vi "FABR-Process Frame.vi"(0 "Runtime in":T2, 7 "SCL in":cluster{T1[]}[](array[cluster]), 9 "AI Waveforms":dbl[](array[numeric]), 11 "error in (no error)":errorcluster, 12 "Reject":dbl, 13 "override":bool) -> (2 "reject fraction":dbl, 3 "Raw":dbl[](array[numeric]), 4 "Runtime out":T2, 8 "SCL out":cluster{T1[]}[](array[cluster]), 10 "update":T1[](array[typedef]), 15 "error out":errorcluster)   [LabVIEW 2020]
uses:
  Typedefs/FABR-Runtime Data.ctl
  Typedefs/FABR-Stimulus Ticket.ctl
  Typedefs/FABR-Stimulus Condition.ctl
  <vilib>/Analysis/baseanly.llb/Mean.vi
  <vilib>/Analysis/baseanly.llb/Mean (DBL).vi
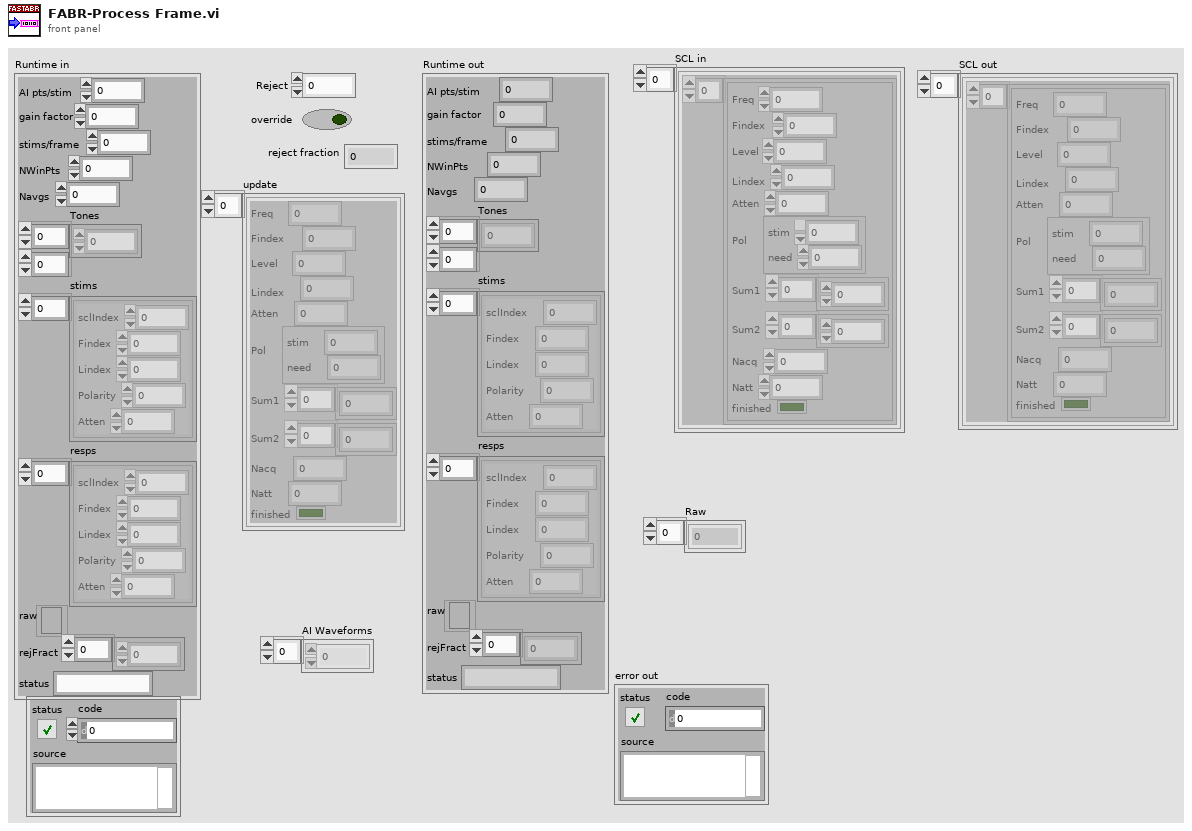
[diagram p1: front panel]
types:
  T1 = typedef "FABR-Stimulus Condition.ctl" = cluster{"Freq":dbl, "Findex":i32, "Level":dbl, "Lindex":i32, "Atten":dbl, "Pol":cluster{"stim":i32, "need":i32}, "Sum1":dbl[], "Sum2":dbl[], "Nacq":i32, "Natt":i32, "finished":bool}
  T2 = typedef "FABR-Runtime Data.ctl" = cluster{"AI pts/stim":i32, "gain factor":dbl, "stims/frame":i32, "NWinPts":i32, "Navgs":i32, "Tones":dbl[][], "stims":T3[], "resps":T3[], "raw":refnum<file>, "rejFract":dbl[], "status":string}
  T3 = typedef "FABR-Stimulus Ticket.ctl" = cluster{"sclIndex":i32, "Findex":i32, "Lindex":i32, "Polarity":i32, "Atten":dbl}
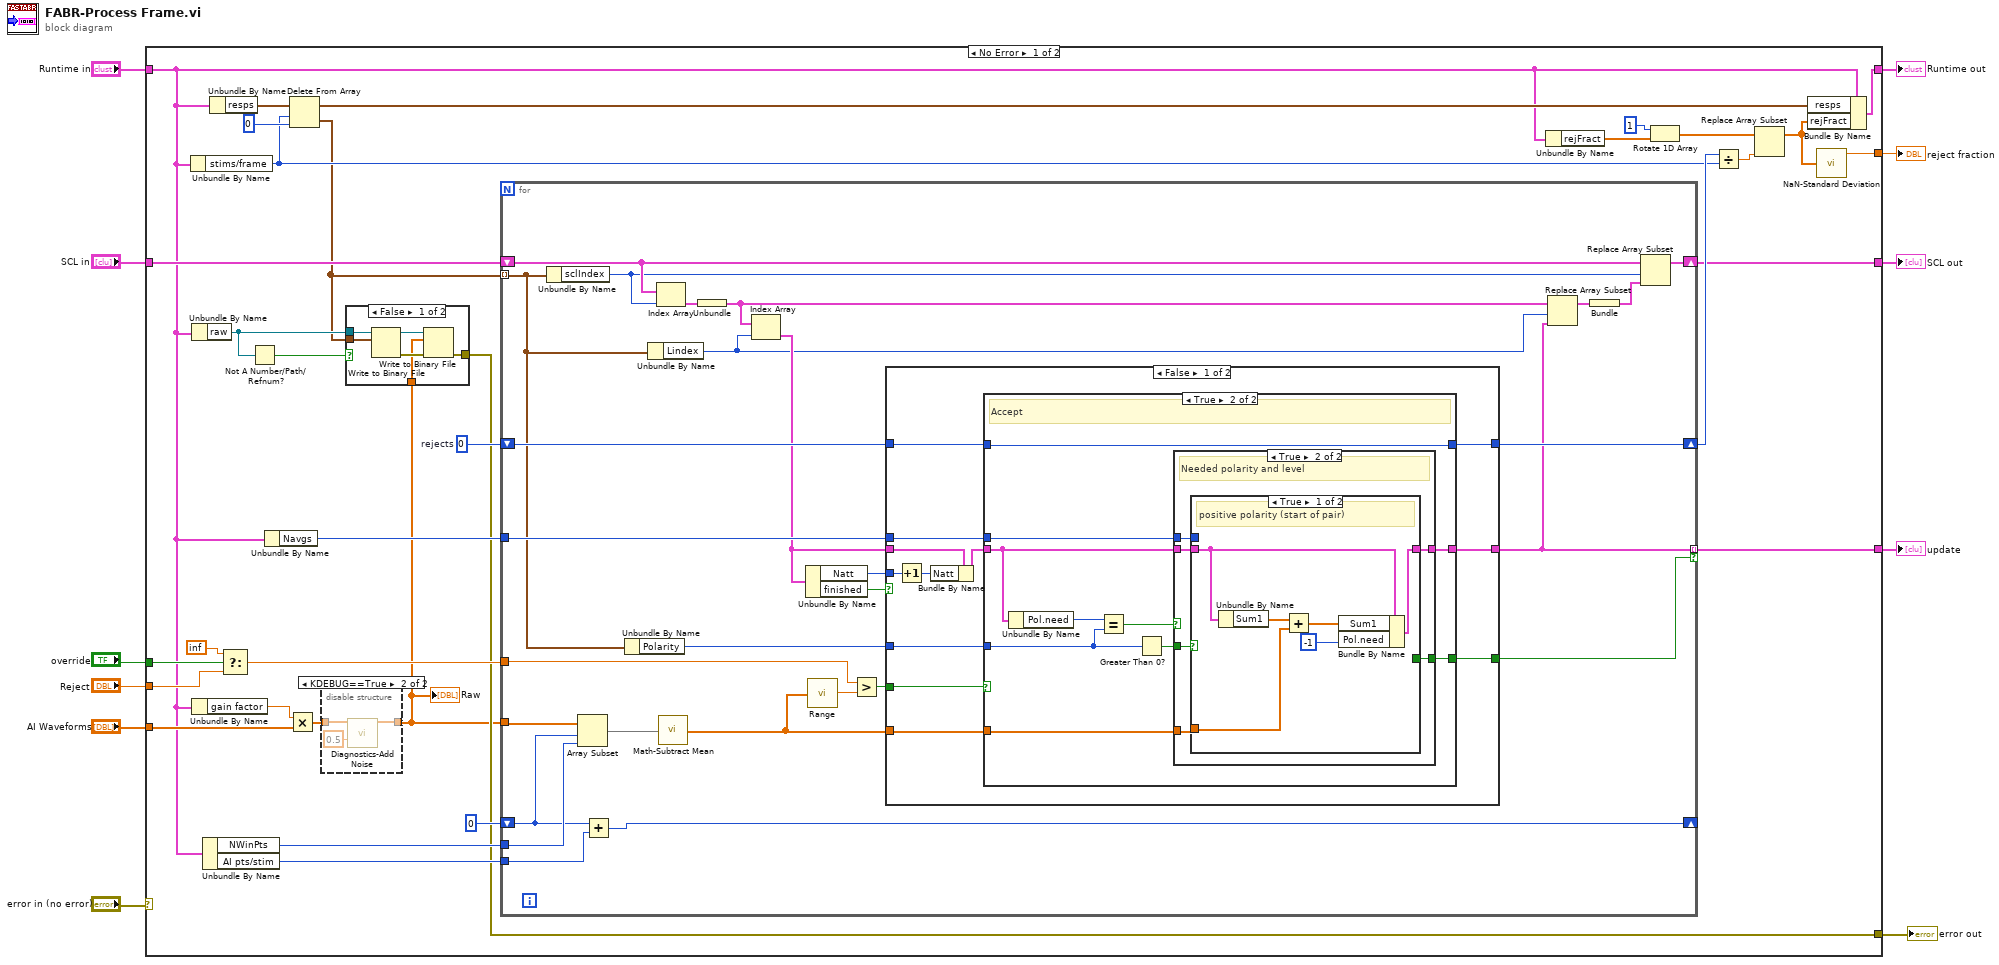
[diagram p0: block diagram]
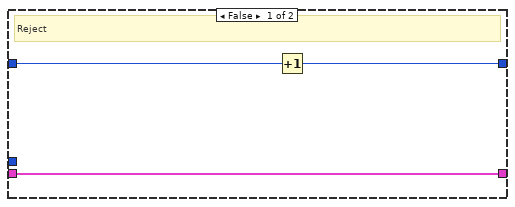
[diagram p4: hidden frame]
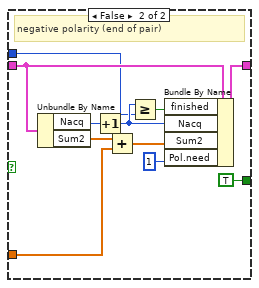
[diagram p6: hidden frame]
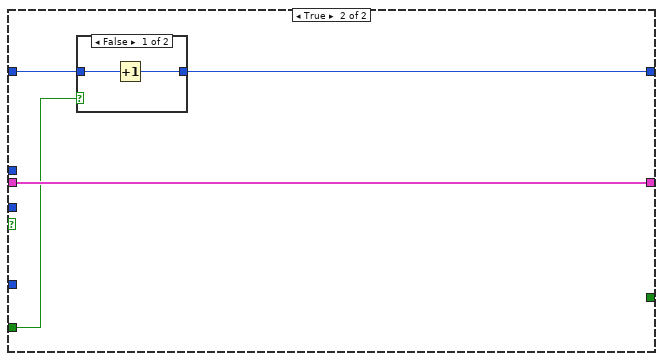
[diagram p7: hidden frame]
diagram:
  n1 = case shown="No Error" "error in (no error)" {
    selector: "error in (no error)" -> [_ w140]
    tunnel: "Runtime in" -> [w20 w139]
    tunnel: "AI Waveforms" -> [w44 _]
    tunnel: "override" -> [w39 _]
    tunnel: "Reject" -> [w38 _]
    tunnel: "SCL in" -> [w31 _]
    tunnel: [w33 _] -> w7
    tunnel: [w32 _] -> w3
    tunnel: [w21 w140] -> w6
    tunnel: [w29 w139] -> w2
    tunnel: [w12 _] -> w1
    frame No Error {
      w35 = 0  # rejects
      n2 = Unbundle By Name(w20) -> ("stims/frame"=w26:i32)
      n3 = Unbundle By Name(w20) -> ("raw"=w23:refnum<file>)
      n4 = Unbundle By Name(w20) -> ("gain factor"=w43:dbl)
      n5 = Unbundle By Name(w20) -> ("NWinPts"=w41:i32, "AI pts/stim"=w40:i32)
      n6 = Unbundle By Name(w20) -> ("resps"=w28:T3[])
      n7 = Select(t=inf, s=w39, f=w38) -> (s? t:f=w36:dbl)
      n8 = Not A Number/Path/Refnum?(number/path/refnum=w23) -> (NaN/Path/Refnum?=w24:bool)
      n9 = Unbundle By Name(w20) -> ("Navgs"=w30:i32)
      n10 = Multiply(x=w43, y=w44) -> (x*y=w17:dbl[])
      n11 = Delete From Array(array=w28, length=w26, index=0) -> (deleted portion=w22:T3[], array with subset deleted=w25:T3[])
      n12 = disable-structure shown="KDEBUG==True" {
        disable-tunnel: w17 -> [w45 w48]
        disable-tunnel: [w45 w47] -> w16
        frame condition #0 (active) {
        }
        frame condition #1 {
          n13 = call "Diagnostics-Add Noise.vi"("Signal"=w48, "Noise RMS"=0.5) -> ("Signal + Noise"=w47:dbl[])  [unwired: 13 in]
        }
      }
      "Raw" <- w16
      n14 = case shown="False" w24 {
        tunnel: w23 -> [w54 _]
        tunnel: w22 -> [w53 _]
        tunnel: w16 -> [w50 _]
        tunnel: [w49 _] -> w21
        frame False {
          n15 = Write to Binary File(file (use dialog)=w54, data=w53) -> (refnum out=w52:refnum<file>, error out=w51:errorcluster)  [unwired: 4 in, 1 out]
          n16 = Write to Binary File(file (use dialog)=w52, data=w50, error in=w51) -> (error out=w49:errorcluster)  [unwired: 3 in, 2 out]
        }
        frame True {
        }
      }
      n17 = for {
        tunnel: w16 -> [w82]
        shift-right: [w78] -> _
        shift-left: 0 -> [w80]
        tunnel: w41 -> [w81]
        tunnel: w40 -> [w79]
        tunnel: w36 -> [w75]
        shift-right: [w72] -> w34
        shift-left: w35 -> [w71]
        shift-right: [w68] -> w32
        shift-left: w31 -> [w69]
        tunnel: [w59] -> w33 mode=indexing if=w67
        tunnel: w30 -> [w64]
        tunnel: w22 -> [w56] mode=indexing
        n18 = Unbundle By Name(w56) -> ("sclIndex"=w66:i32)
        n19 = Array Subset(array=w82, index=w80, length=w81) -> (w77:dbl[])
        n20 = Add(x=w80, y=w79) -> (x+y=w78:i32)
        n21 = Unbundle By Name(w56) -> ("Polarity"=w65:i32)
        n22 = Unbundle By Name(w56) -> ("Lindex"=w60:i32)
        n23 = Index Array(array=w69, index=w66) -> (element=w63:cluster{T1[]})
        n24 = call "Math-Subtract Mean.vi"("Y"=w77) -> ("Y - mean(Y)"=w73:dbl[])  [unwired: 4 in]
        n25 = Unbundle(w63) -> (w61:T1[])
        n26 = Index Array(array=w61, index=w60) -> (element=w62:T1)
        n27 = Unbundle By Name(w62) -> ("Natt"=w70:i32, "finished"=w55:bool)
        n28 = call "Range.vi"("Array"=w73) -> ("Range"=w76:dbl)
        n29 = Greater?(x=w75, y=w76) -> (0:w74:bool)
        n30 = case shown="False" w55 {
          tunnel: w74 -> [w94 w134]
          tunnel: w73 -> [w93 _]
          tunnel: [w92 w132] -> w72
          tunnel: w71 -> [w91 w133]
          tunnel: w70 -> [w90 _]
          tunnel: [w87 _] -> w67
          tunnel: w65 -> [w86 _]
          tunnel: w64 -> [w85 _]
          tunnel: w62 -> [w84 w135]
          tunnel: [w83 w135] -> w59
          frame False {
            n31 = Increment(x=w90) -> (x+1=w89:i32)
            n32 = Bundle By Name(cluster=w84, "Natt"=w89) -> (w88:T1)
            n33 = case shown="True" w94 {
              tunnel: w93 -> [_ w105]
              tunnel: [w96 w107] -> w92
              tunnel: w91 -> [w97 w107]
              tunnel: w88 -> [w95 w99]
              tunnel: [w95 w104] -> w83
              tunnel: [_ w103] -> w87
              tunnel: w86 -> [_ w101]
              tunnel: w85 -> [_ w98]
              frame False {
                # "Reject"
                n34 = Increment(x=w97) -> (x+1=w96:i32)
              }
              frame True {
                # "Accept"
                n35 = Unbundle By Name(w99) -> ("Pol.need"=w102:i32)
                n36 = Equal?(x=w102, y=w101) -> (x = y?=w100:bool)
                n37 = Greater Than 0?(x=w101) -> (x > 0?=w106:bool)
                n38 = case shown="True" w100 {
                  tunnel: w106 -> [_ w114]
                  tunnel: w105 -> [_ w113]
                  tunnel: w99 -> [w108 w112]
                  tunnel: [w108 w111] -> w104
                  tunnel: [_ w110] -> w103
                  tunnel: w98 -> [_ w109]
                  frame False {
                    # "Wrong polarity or level"
                  }
                  frame True {
                    # "Needed polarity and level"
                    n39 = case shown="True" w114 {
                      tunnel: w112 -> [w117 w129]
                      tunnel: w113 -> [w119 w130]
                      tunnel: [w116 w126] -> w111
                      tunnel: [_ TRUE] -> w110
                      tunnel: w109 -> [_ w121]
                      frame True {
                        # "positive polarity (start of pair)"
                        n40 = Unbundle By Name(w117) -> ("Sum1"=w120:dbl[])
                        n41 = Add(x=w120, y=w119) -> (x+y=w118:dbl[])
                        n42 = Bundle By Name(cluster=w117, "Sum1"=w118, "Pol.need"=-1 ("awaiting")) -> (w116:T1)
                      }
                      frame False {
                        # "negative polarity (end of pair)"
                        n43 = Unbundle By Name(w129) -> ("Nacq"=w127:i32, "Sum2"=w131:dbl[])
                        n44 = Increment(x=w127) -> (x+1=w122:i32)
                        n45 = Add(x=w131, y=w130) -> (x+y=w128:dbl[])
                        n46 = Greater Or Equal?(x=w122, y=w121) -> (x >= y?=w123:bool)
                        n47 = Bundle By Name(cluster=w129, "finished"=w123, "Nacq"=w122, "Sum2"=w128, "Pol.need"=1 ("awaiting")) -> (w126:T1)
                      }
                    }
                  }
                }
              }
            }
          }
          frame True {
            n48 = case shown="False" w134 {
              tunnel: w133 -> [w137 w138]
              tunnel: [w136 w138] -> w132
              frame False {
                n49 = Increment(x=w137) -> (x+1=w136:i32)
              }
              frame True {
              }
            }
          }
        }
        n50 = Replace Array Subset(array=w61, new element=w59, index=w60) -> (w58:T1[])
        n51 = Bundle(w58) -> (w57:cluster{T1[]})  [unwired: 1 in]
        n52 = Replace Array Subset(array=w69, new element=w57, index=w66) -> (w68:cluster{T1[]}[])
      }
      n53 = Unbundle By Name(w20) -> ("rejFract"=w19:dbl[])
      n54 = Rotate 1D Array(1:w19, 2:1 ("n")) -> (0:w15:dbl[])
      n55 = Divide(x=w34, y=w26) -> (x/y=w13:dbl)
      n56 = Replace Array Subset(array=w15, new element=w13) -> (w14:dbl[])  [unwired: 1 in]
      n57 = Bundle By Name(cluster=w20, "resps"=w25, "rejFract"=w14) -> (w29:T2)
      n58 = call "NaN-Standard Deviation.vi"("Array"=w14) -> ("mean"=w12:dbl)  [unwired: 3 in, 1 out]
    }
    frame Error {
    }
  }
  "error out" <- w6
  "Runtime out" <- w2
  "update" <- w7
  "reject fraction" <- w1
  "SCL out" <- w3
